vi "test Set and Get Possible Endpoints.vi"(8 "error in (no error)":errorcluster, 11 "TestCase in":refnum<class "SLSC Switch Scripting Unit Tests.lvclass">) -> (0 "error out":errorcluster, 3 "TestCase out":refnum<class "SLSC Switch Scripting Unit Tests.lvclass">)   [LabVIEW 2017, in "SLSC Switch Scripting Unit Tests.lvclass"]
uses:
  SLSC Switch Scripting Unit Tests.lvclass
  Shared/Routing and Faulting Hardware API/Types/Possible Connections for Endpoint.ctl
  SLSC Switch Scripting Unit Tests.lvclass/SLSC Switch Scripting Unit Tests.ctl
  Custom Device/Find All SLSC Switch Custom Devices.vi
  <vilib>/addons/_JKI Toolkits/VI Tester/TestCase.llb/TestCase.lvclass
  SLSC Switch Scripting.lvlib
  Shared/Routing and Faulting Hardware API/Routing and Faulting Hardware API.lvlib
  C:/Program Files (x86)/National Instruments/LabVIEW 2017/vi.lib/addons/_JKI Toolkits/VI Tester/TestCase.llb/TestCase.lvclass
panel:
  in  "Save?":bool
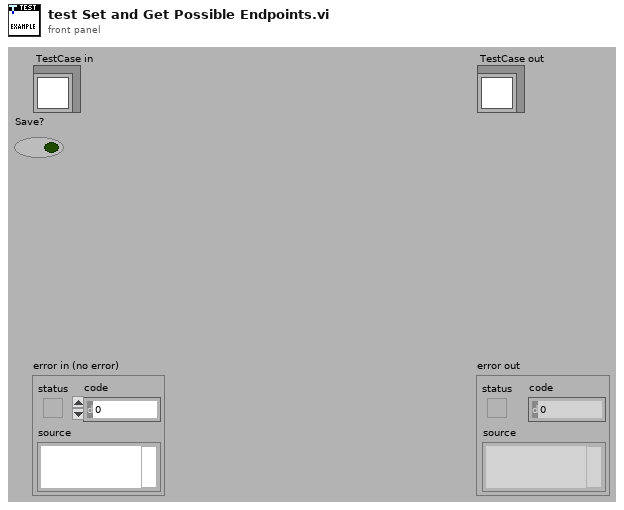
[diagram p1: front panel]
types:
  T1 = typedef "Routing and Faulting Hardware API.lvlib/Possible Connections for Endpoint.ctl" = cluster{"Source":string, "Destinations":string[]}
  T2 = typedef "Custom Device API.lvlib/Custom Device Item Ref.ctl" = u64
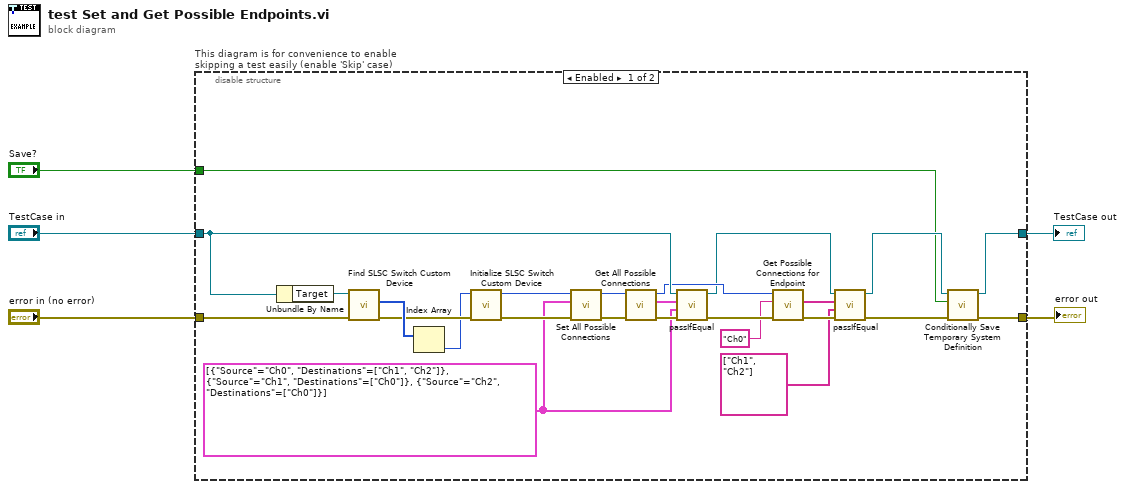
[diagram p0: block diagram]
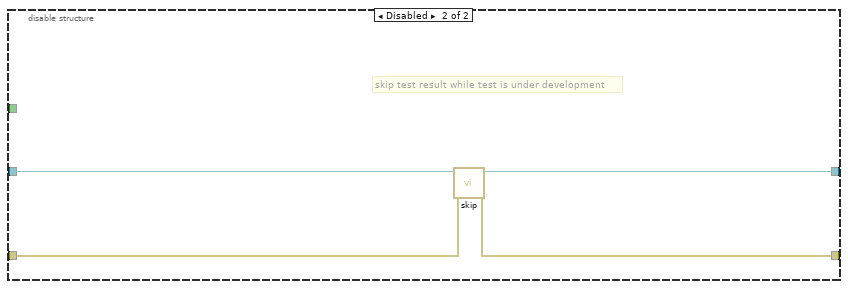
[diagram p2: hidden frame]
diagram:
  n1 = disable-structure "This diagram is for convenience to enable skipping a test easily (enable 'Skip' case)" shown="Enabled" {
    disable-tunnel: "TestCase in" -> [w20 w34]
    disable-tunnel: [w14 w32] -> w2
    disable-tunnel: [w13 w33] -> w4
    disable-tunnel: "error in (no error)" -> [w26 w31]
    disable-tunnel: "Save?" -> [w6 _]
    frame Enabled {
      w18 = T1[] [{"Source"="Ch0", "Destinations"=["Ch1", "Ch2"]}, {"Source"="Ch1", "Destinations"=["Ch0"]}, {"Source"="Ch2", "Destinations"=["Ch0"]}] ("Possible Connections")
      n2 = Unbundle By Name(w20) -> ("Target"=w27:refnum<k24>)
      n3 = call-poly "Find SLSC Switch Custom Device.vi"("error in (no error)"=w26, "Target in"=w27) -> ("error out"=w29:errorcluster, "SLSC Switch Custom Device Ref IDs"=w30:T2[])  [unwired: 7 in, 1 out]
      n4 = Index Array(array=w30) -> (element=w28:T2)  [unwired: 1 in]
      n5 = call "Initialize SLSC Switch Custom Device.vi"("error in (no error)"=w29, "SLSC Switch Custom Device Ref in"=w28) -> ("error out"=w24:errorcluster, "SLSC Switch Custom Device Ref out"=w25:T2)  [unwired: 7 in, 1 out]
      n6 = call "Set All Possible Connections.vi"("error in (no error)"=w24, "Possible Connections"=w18, "Hardware Ref in"=w25) -> ("error out"=w23:errorcluster, "Hardware Ref out"=w22:T2)  [unwired: 7 in]
      n7 = call "Get All Possible Connections.vi"("error in (no error)"=w23, "Hardware Ref in"=w22) -> ("error out"=w21:errorcluster, "Possible Connections"=w19:T1[], "Hardware Ref out"=w16:T2)  [unwired: 7 in]
      n8 = call-dynamic "passIfEqual.vi"("error in (no error)"=w21, "y"=w18, "x"=w19, "TestCase in"=w20) -> ("error out"=w17:errorcluster, "TestCase out"=w11:refnum<class "SLSC Switch Scripting Unit Tests.lvclass">)  [unwired: 6 in]
      n9 = call "Get Possible Connections for Endpoint.vi"("error in (no error)"=w17, "Endpoint"="Ch0", "Hardware Ref in"=w16) -> ("error out"=w9:errorcluster, "Possible Connections"=w12:string[])  [unwired: 6 in, 1 out]
      n10 = call-dynamic "passIfEqual.vi"("error in (no error)"=w9, "y"=string[] ["Ch1", "Ch2"] ("Destinations"), "x"=w12, "TestCase in"=w11) -> ("error out"=w8:errorcluster, "TestCase out"=w10:refnum<class "SLSC Switch Scripting Unit Tests.lvclass">)  [unwired: 6 in]
      n11 = call "Conditionally Save Temporary System Definition.vi"("error in (no error)"=w8, "Save?"=w6, "Test Case"=w10) -> ("error out"=w13:errorcluster, "Test Case"=w14:refnum<class "SLSC Switch Scripting Unit Tests.lvclass">)  [unwired: 6 in, 1 out]
    }
    frame Disabled {
      # "skip test result while test is under development"
      n12 = call <vilib>:"skip.vi"("error in (no error)"=w31, "TestCase in"=w34) -> ("error out"=w33:errorcluster, "TestCase out"=w32:refnum<class "SLSC Switch Scripting Unit Tests.lvclass">)  [unwired: 8 in]
    }
  }
  "error out" <- w4
  "TestCase out" <- w2
